vi "Temp to % v1.vi"(1 "Minimum Temp":dbl format="%.2f", 2 "Input Temp":dbl format="%.2f", 3 "Maximum Temp":dbl=100.0 format="%.2f") -> (0 "Output Percentage":dbl format="%.2f")   [LabVIEW 2012]
panel:
  # "Temp to %"
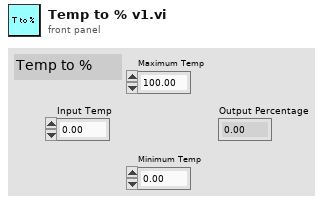
[diagram p1: front panel]
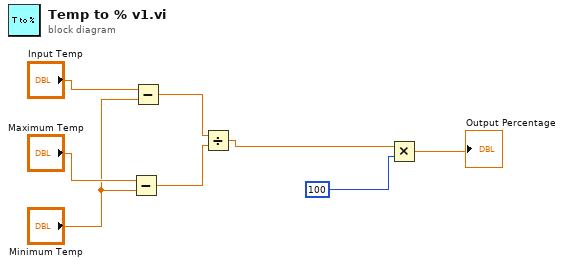
[diagram p0: block diagram]
diagram:
  n1 = Subtract(x="Maximum Temp", y="Minimum Temp") -> (x-y=w4:dbl)
  n2 = Subtract(x="Input Temp", y="Minimum Temp") -> (x-y=w5:dbl)
  n3 = Divide(x=w5, y=w4) -> (x/y=w3:dbl)
  n4 = Multiply(x=w3, y=100) -> (x*y=→"Output Percentage":dbl)
